vi "test1.vi"() -> ()   [LabVIEW 2026]
doc: "Trial"
panel:
  out "x+y":dbl
  in  "x":dbl
  in  "y":dbl
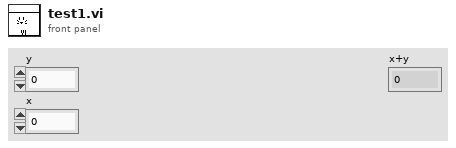
[diagram p1: front panel]
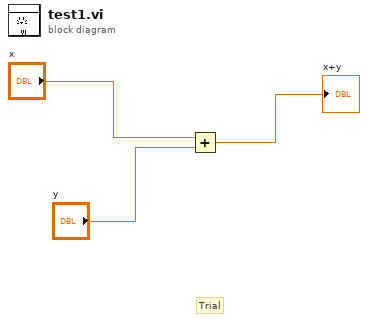
[diagram p0: block diagram]
diagram:
  # "Trial"
  n1 = Add(x="x", y="y") -> (x+y=→"x+y":dbl)
